vi "Dequeue Master and Local.vi"(8 "error in (no error)":errorcluster, 9 "Instrument Name":string, 10 "Master":refnum<queue>, 11 "UI":refnum<queue>) -> (0 "error out":errorcluster, 1 "Message Data":variant, 2 "Message":string, 3 "UI out":refnum<queue>)   [LabVIEW 2014, in "MeasurementControl Message Queue.lvlib"]
uses:
  MeasurementControl Message Queue.lvlib
  Message Cluster.ctl
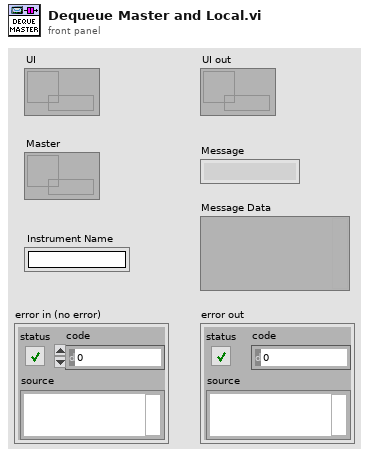
[diagram p1: front panel]
types:
  T1 = typedef "MeasurementControl Message Queue.lvlib/Message Cluster.ctl" = cluster{"Message":string, "Message Data":variant}
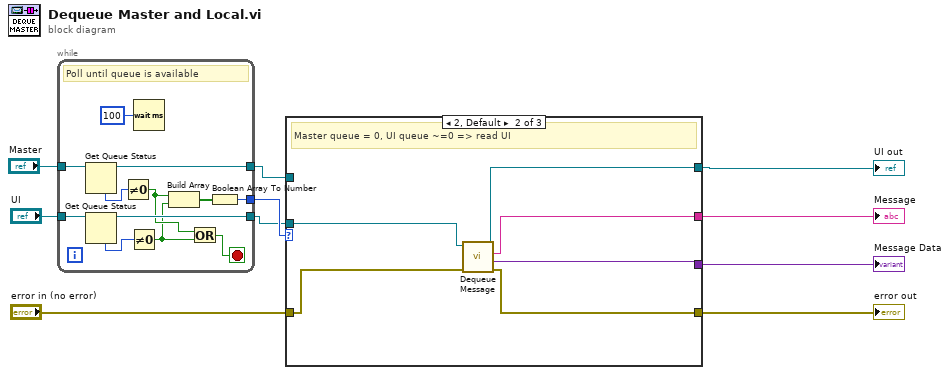
[diagram p0: block diagram]
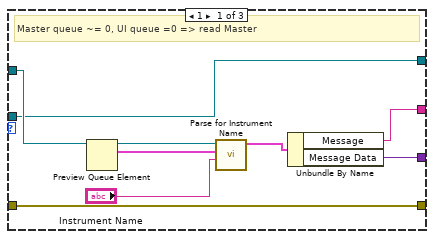
[diagram p2: hidden frame]
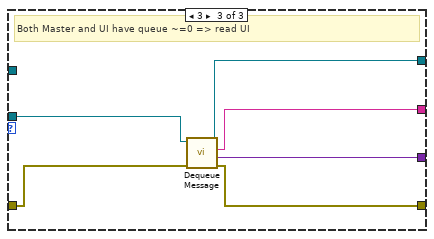
[diagram p3: hidden frame]
diagram:
  n1 = while {
    tunnel: "UI" -> [w22]
    tunnel: "Master" -> [w19]
    tunnel: [w17] -> w8
    tunnel: [w16] -> w7
    tunnel: [w15] -> w6
    stop <- w13 stop-if-true
    # "Poll until queue is available"
    n2 = Get Queue Status(queue=w19) -> (queue out=w16:refnum<queue>, # elements in queue=w20:i32)  [unwired: 2 in, 6 out]
    n3 = Get Queue Status(queue=w22) -> (queue out=w15:refnum<queue>, # elements in queue=w21:i32)  [unwired: 2 in, 6 out]
    n4 = Not Equal To 0?(x=w20) -> (x != 0?=w12:bool)
    n5 = Not Equal To 0?(x=w21) -> (x != 0?=w11:bool)
    n6 = Wait (ms)(milliseconds to wait=u32 100) -> ()  [unwired: 1 out]
    n7 = Build Array(w12, w11) -> (w18:bool[])
    n8 = Or(x=w12, y=w11) -> (x .or. y?=w13:bool)
    n9 = Boolean Array To Number(Boolean array=w18) -> (number=w17:u32)
  }
  n10 = case shown="2, Default" w8 {
    tunnel: w7 -> [w28 _ _]
    tunnel: w6 -> [w23 w33 w38]
    tunnel: "error in (no error)" -> [w29 w34 w43]
    tunnel: [w23 w32 w39] -> w4
    tunnel: [w31 w37 w40] -> w3
    tunnel: [w30 w36 w41] -> w2
    tunnel: [w29 w35 w42] -> w1
    frame 1 {
      # "Master queue ~= 0, UI queue =0 => read Master"
      n11 = Preview Queue Element(queue=w28) -> (queue out=w27:refnum<queue>, element=w25:T1)  [unwired: 2 in, 2 out]
      n12 = call "Parse for Instrument Name.vi"("Instrument Name"="Instrument Name", "Message In"=w25, "Message Queue"=w27) -> ("Message Out"=w24:T1)  [unwired: 8 in]
      n13 = Unbundle By Name(w24) -> ("Message"=w31:string, "Message Data"=w30:variant)
    }
    frame 2, Default {
      # "Master queue = 0, UI queue ~=0 => read UI"
      n14 = call "Dequeue Message.vi"("error in (no error)"=w34, "Message Queue"=w33) -> ("error out"=w35:errorcluster, "Message Data"=w36:variant, "Message"=w37:string, "dup Message Queue"=w32:refnum<queue>)  [unwired: 6 in]
    }
    frame 3 {
      # "Both Master and UI have queue ~=0 => read UI"
      n15 = call "Dequeue Message.vi"("error in (no error)"=w43, "Message Queue"=w38) -> ("error out"=w42:errorcluster, "Message Data"=w41:variant, "Message"=w40:string, "dup Message Queue"=w39:refnum<queue>)  [unwired: 6 in]
    }
  }
  "error out" <- w1
  "Message Data" <- w2
  "Message" <- w3
  "UI out" <- w4
